vi "I2C Ultrasonic Sensor.vi"(6 "I2C Communication Values":T1 {"Command 2" format="%x"; "Command 1" format="%x"; "Address" format="%x"}, 7 "FPGA VI Reference In":refnum<k20>) -> (2 "Distance":u32 format="%b")   [LabVIEW 2013]
uses:
  <vilib>/rvi/interface/common/niFpgaWaitOnOcc.vi
  <vilib>/Utility/error.llb/Error Cluster From Error Code.vi
  <vilib>/rvi/errors/niLvFpgaAdjustHostInterfaceError.vi
  <vilib>/rvi/interface/nirviReadWriteControl/nirviReadWriteControl.xnode
  <vilib>/rvi/interface/Simulation/niFpgaSimulationCallBeginRW.vi
  NiFpgaLv.dll
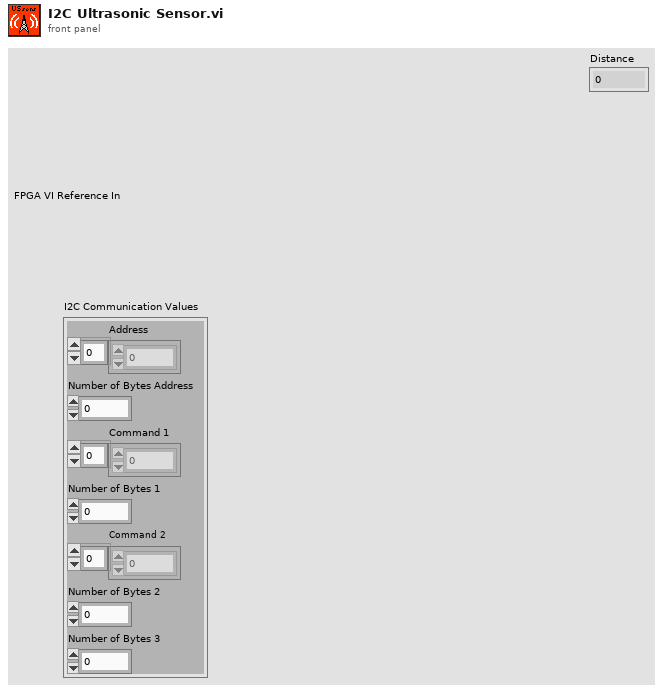
[diagram p1: front panel]
types:
  T1 = cluster{"Address":i8[], "Number of Bytes Address":i8, "Command 1":i8[], "Number of Bytes 1":i8, "Command 2":i8[], "Number of Bytes 2":i8, "Number of Bytes 3":i8}
  T2 = cluster{"Address":i8[], "Number of Bytes Address":i8, "Command 1":i8[], "Number of Bytes 1":i8, "Command 2":i8[], "Number of Bytes 2":i8, "Number of Bytes 3":i8, bool}
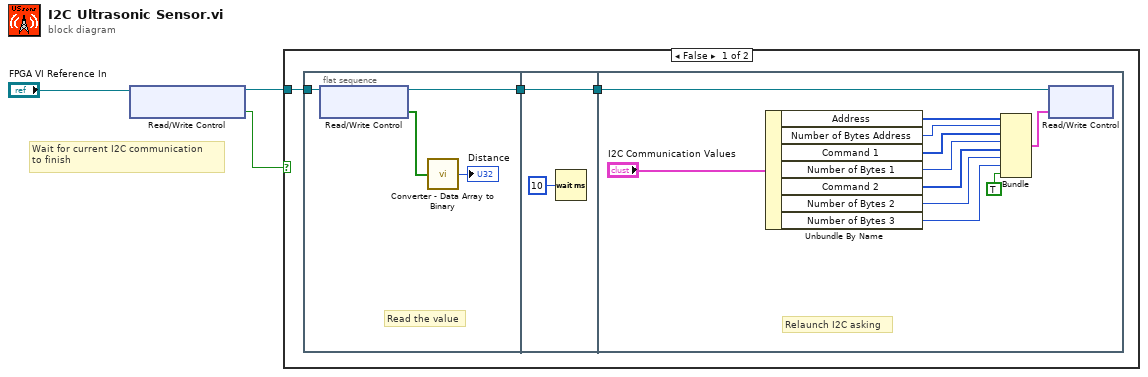
[diagram p0: block diagram]
diagram:
  # "Wait for current I2C communication\nto finish"
  n1 = xnode "Read/Write Control"("FPGA VI Reference In"="FPGA VI Reference In") -> ("FPGA VI Reference Out"=w3:refnum<k20>, "I2C FPGA Running"=w2:bool)  [unwired: 1 in, 1 out]
  n2 = case shown="False" w2 {
    tunnel: w3 -> [w6 _]
    frame False {
      n3 = flat-sequence {
        tunnel: w6 -> [w8]
        tunnel: [w7] -> w4
        tunnel: [w12] -> w5
        tunnel: w4 -> [w12]
        tunnel: w5 -> [w23]
        frame #0 {
          # "Read the value"
          n4 = xnode "Read/Write Control"("FPGA VI Reference In"=w8) -> ("FPGA VI Reference Out"=w7:refnum<k20>, "Data bit array"=w10:bool[])  [unwired: 1 in, 1 out]
          n5 = call "Converter - Data Array to Binary.vi"("Data bit array"=w10) -> ("Value"=→"Distance":u32)
        }
        frame #1 {
          n6 = Wait (ms)(milliseconds to wait=u32 10) -> ()  [unwired: 1 out]
        }
        frame #2 {
          # "Relaunch I2C asking"
          n7 = Unbundle By Name("I2C Communication Values") -> ("Address"=w19:i8[], "Number of Bytes Address"=w18:i8, "Command 1"=w17:i8[], "Number of Bytes 1"=w16:i8, "Command 2"=w15:i8[], "Number of Bytes 2"=w14:i8, "Number of Bytes 3"=w13:i8)
          n8 = Bundle("Address"=w19, "Number of Bytes Address"=w18, "Command 1"=w17, "Number of Bytes 1"=w16, "Command 2"=w15, "Number of Bytes 2"=w14, "Number of Bytes 3"=w13, TRUE) -> (w22:T2)  [unwired: 1 in]
          n9 = xnode "Read/Write Control"("FPGA VI Reference In"=w23, "I2C Read"=w22) -> ()  [unwired: 1 in, 2 out]
        }
      }
    }
    frame True {
    }
  }
